vi "H5ErrorHandler2.vi"(4 "error in (no error)":errorcluster, 6 "Error code Offset":i32=402760) -> (0 "error out":errorcluster)   [LabVIEW 2017]
panel:
  # "LVHDF5 Toolkit\nCopyright (c) 2005-2013 by Jason D. Sommerville\nCopyright (c) 2014 by UPVI, LLC.\n\nThis use and distribution of this file is governed by the terms found in \nLICENSE.txt distributed with this toolkit and installed at\n <user.lib>\\_lvhdf5\\LICENSE.txt"
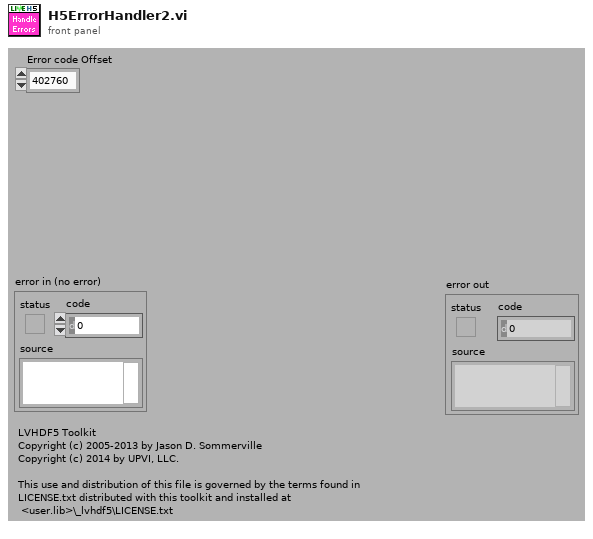
[diagram p1: front panel]
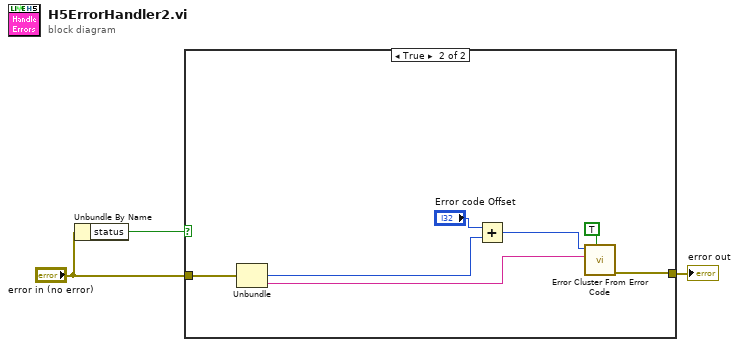
[diagram p0: block diagram]
diagram:
  n1 = Unbundle By Name("error in (no error)") -> ("status"=w1:bool)
  n2 = case shown="True" w1 {
    tunnel: [w4 w11] -> w3
    tunnel: "error in (no error)" -> [w4 w7]
    frame False {
    }
    frame True {
      n3 = Unbundle(w7) -> ("code"=w6:i32, "source"=w5:string)  [unwired: 1 out]
      n4 = Add(x="Error code Offset", y=w6) -> (x+y=w9:i32)
      n5 = call <vilib>:"Error Cluster From Error Code.vi"("show call chain? (False)"=TRUE, "error message (\"\")"=w5, "error code (0)"=w9) -> ("error out"=w11:errorcluster)  [unwired: 6 in]
    }
  }
  "error out" <- w3
